vi "Instrument Manager Loop.vi"(8 "System Control":refnum<queue>, 11 "Instrument Manager":refnum<queue>) -> (0 "error out":errorcluster)   [LabVIEW 2020, in "ChromTech Next Gen Compensator Pump.lvlib" / "Instrument Manager.lvlib"]
uses:
  Instrument Manager/Instrument Manager.lvlib
  support/Message Queue/Message Cluster.ctl
  Instrument Manager/Instrument State.ctl
  <vilib>/Utility/error.llb/Error Cluster From Error Code.vi
  <vilib>/ErrorRing/Error Ring.xnode
  support/Message Queue/Message Queue.lvlib
  ChromTech Next Gen Compensator Pump.lvlib
  <instrlib>/RxnRover/ChromtechNextGenDriver/ChromTech MX-Class Drivers.lvlib
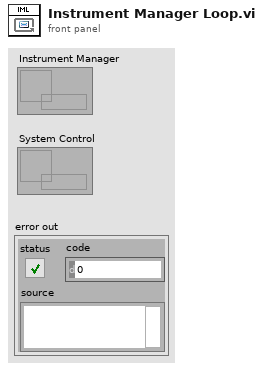
[diagram p1: front panel]
types:
  T1 = typedef "ChromTech Next Gen Compensator Pump.lvlib/Instrument Manager.lvlib/Instrument State.ctl" = cluster{"VISA Resource":refnum<visa-resource-name>, "Flow Rate":dbl, "Running":bool, "Running Since":timestamp, "Pressure Data Point":cluster{"Time Stamp":timestamp, "Value":dbl}, "Upper Pressure Fault":bool, "Lower Pressure Fault":bool, "Motor Stall Fault":bool, "Sampling Rate (sec/sample)":dbl, "Retry Attempts":i32, "Fast Comms":bool, "Total Flow Rate":dbl, "Other Flow Rate":dbl}
  T2 = cluster{"seconds since 1Jan1904":timestamp, "Pressure":dbl}
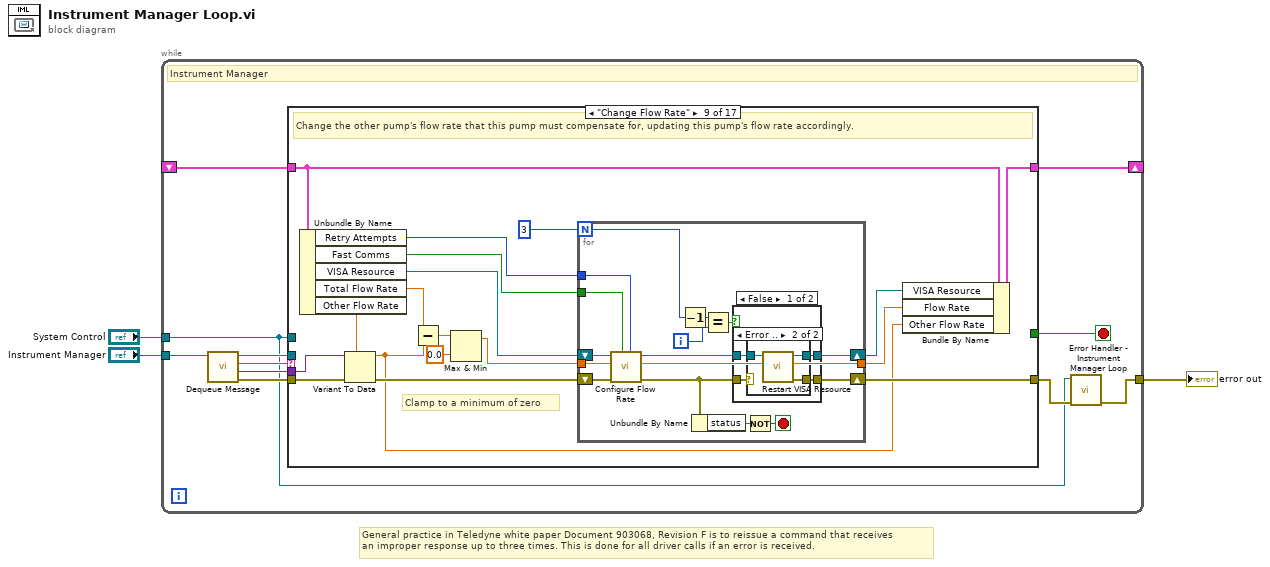
[diagram p0: block diagram]
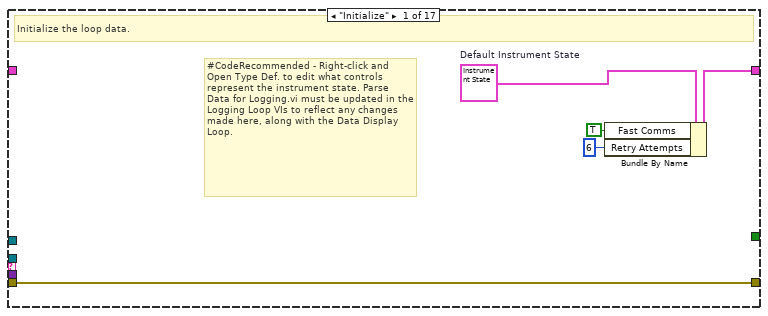
[diagram p2: hidden frame]
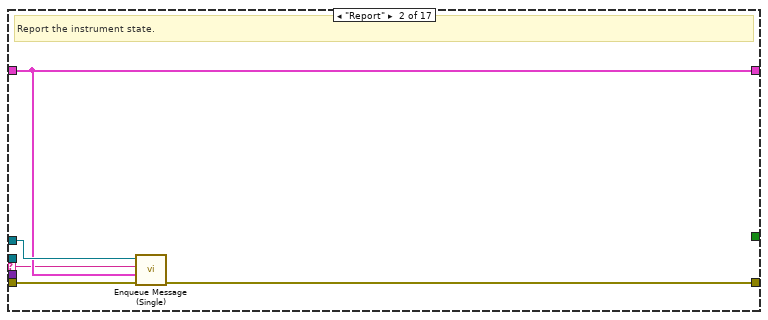
[diagram p3: hidden frame]
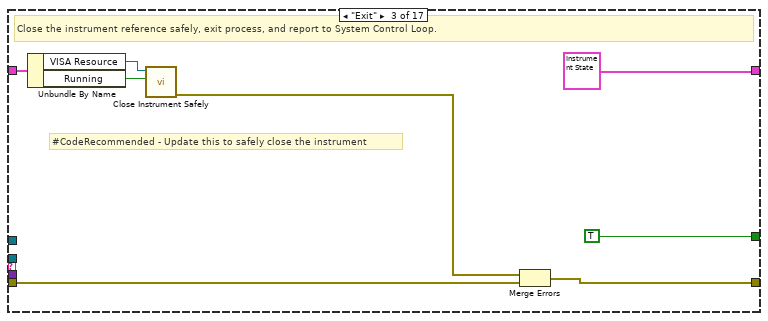
[diagram p4: hidden frame]
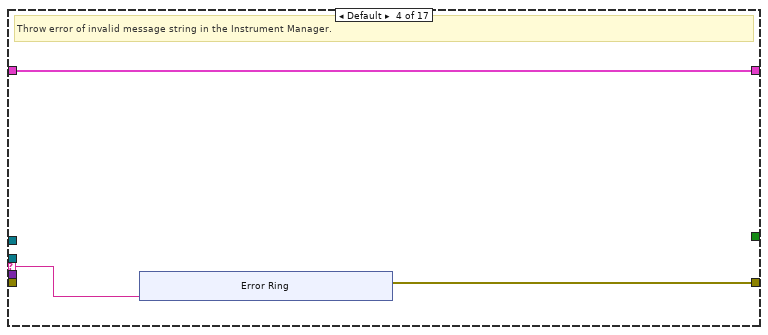
[diagram p5: hidden frame]
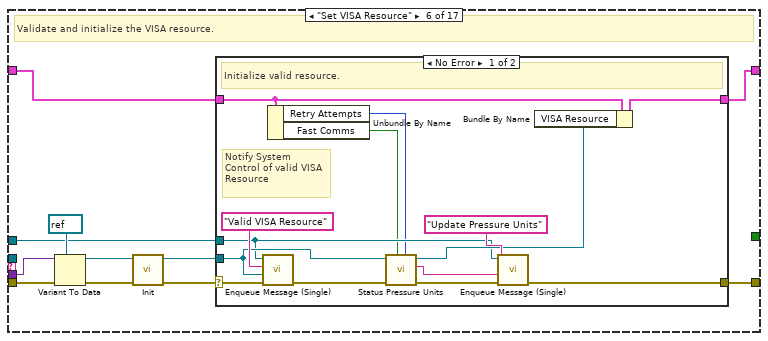
[diagram p7: hidden frame]
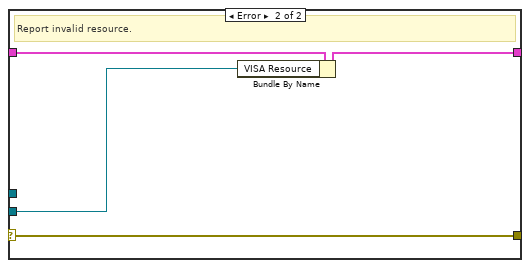
[diagram p8: hidden frame]
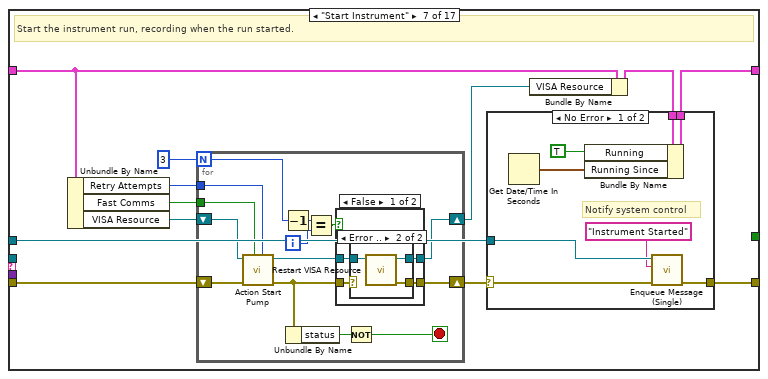
[diagram p9: hidden frame]
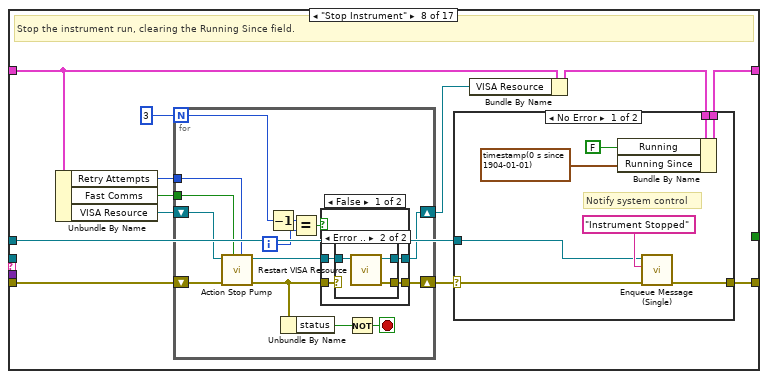
[diagram p13: hidden frame]
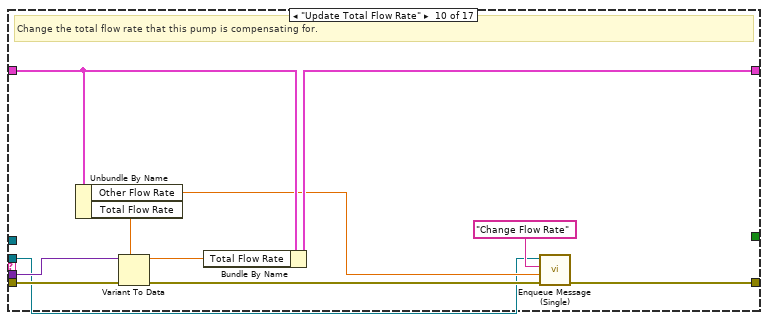
[diagram p19: hidden frame]
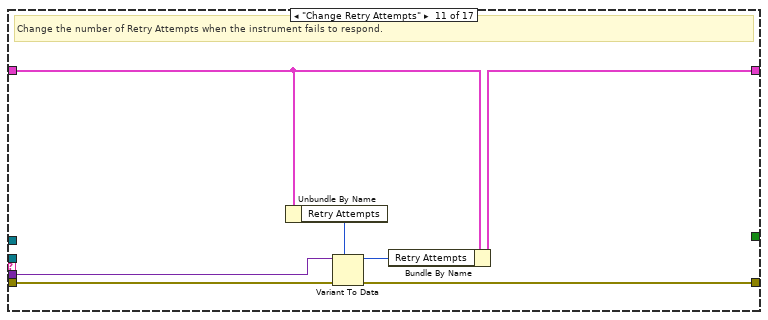
[diagram p20: hidden frame]
diagram:
  # "General practice in Teledyne white paper Document 903068, Revision F is to reissue a command that receives\nan improper response up to three times. This is done for all driver calls if an error is received."
  n1 = while {
    tunnel: "Instrument Manager" -> [w14]
    tunnel: "System Control" -> [w4]
    tunnel: [w8] -> w1
    shift-right: [w6] -> _
    shift-left: _ -> [w7]
    stop <- w5 stop-if-true
    # "Instrument Manager"
    n2 = call "Dequeue Message.vi"("Message Queue"=w14) -> ("error out"=w10:errorcluster, "Message Data"=w11:variant, "Message"=w13:string, "dup Message Queue"=w12:refnum<queue>)  [unwired: 7 in]
    n3 = case shown="\"Change Flow Rate\"" w13 {
      selector: w13 -> [_ w20 _ w34 _ _ _ _ _ _ _ _ _ _ _ _ _]
      tunnel: w12 -> [_ _ _ _ _ _ _ _ _ w213 _ _ _ _ _ _ _]
      tunnel: w4 -> [_ w23 _ _ _ w45 w84 w131 _ _ _ _ _ _ _ _ _]
      tunnel: w11 -> [_ _ _ _ _ w52 _ _ w184 w222 w229 w236 _ _ _ _ _]
      tunnel: w10 -> [w18 w24 w27 _ w43 w51 w82 w129 w175 w219 w225 w232 w240 w249 w284 w324 w365]
      tunnel: [w18 w22 w26 w33 w43 w55 w85 w132 w181 w215 w224 w231 w240 w248 w283 w322 w358] -> w9
      tunnel: w7 -> [_ w21 w32 w35 w44 w54 w81 w127 w183 w221 w228 w235 w239 w247 w285 w321 w362]
      tunnel: [w17 w21 T1 {"VISA Resource"="", "Flow Rate"=0.0, "Running"=FALSE, "Running Since"=timestamp(0 s since 1904-01-01), "Pressure Data Point"={"Time Stamp"=timestamp(0 s since 1904-01-01), "Value"=0.0}, "Upper Pressure Fault"=FALSE, "Lower Pressure Fault"=FALSE, "Motor Stall Fault"=FALSE, "Sampling Rate (sec/sample)"=0.0, "Retry Attempts"=0, "Fast Comms"=FALSE, "Total Flow Rate"=0.0, "Other Flow Rate"=0.0} w35 w44 w53 w83 w130 w185 w223 w230 w237 w239 w250 w288 w323 w364] -> w6
      tunnel: [_ _ TRUE _ _ _ _ _ _ _ _ _ _ _ _ _ _] -> w5
      frame "Initialize" {
        w19 = T1 {"VISA Resource"="", "Flow Rate"=0.0, "Running"=FALSE, "Running Since"=timestamp(0 s since 1904-01-01), "Pressure Data Point"={"Time Stamp"=timestamp(0 s since 1904-01-01), "Value"=0.0}, "Upper Pressure Fault"=FALSE, "Lower Pressure Fault"=FALSE, "Motor Stall Fault"=FALSE, "Sampling Rate (sec/sample)"=0.0, "Retry Attempts"=0, "Fast Comms"=FALSE, "Total Flow Rate"=0.0, "Other Flow Rate"=0.0}  # Default Instrument State
        # "#CodeRecommended - Right-click and Open Type Def. to edit what controls represent the instrument state. Parse Data for Logging.vi must be updated in the Logging Loop VIs to reflect any changes made here, along with the Data Display Loop."
        # "Initialize the loop data."
        n4 = Bundle By Name(cluster=w19, "Fast Comms"=TRUE, "Retry Attempts"=6) -> (w17:T1)
      }
      frame "Report" {
        # "Report the instrument state."
        n5 = call "Enqueue Message (Single).vi"("error in (no error)"=w24, "Message Data"=w21, "Message"=w20, "Message Queue"=w23) -> ("error out"=w22:errorcluster)  [unwired: 6 in, 1 out]
      }
      frame "Exit" {
        # "#CodeRecommended - Update this to safely close the instrument"
        # "Close the instrument reference safely, exit process, and report to System Control Loop."
        n6 = Unbundle By Name(w32) -> ("VISA Resource"=w30:refnum<visa-resource-name>, "Running"=w31:bool)
        n7 = call "Close Instrument Safely.vi"("Running (F)"=w31, "VISA Refnum in"=w30) -> ("error out"=w25:errorcluster)  [unwired: 9 in]
        n8 = Merge Errors(w25, w27) -> (w26:errorcluster)
      }
      frame Default {
        # "Throw error of invalid message string in the Instrument Manager."
        n9 = xnode "Error Ring"("parameter 0"=w34) -> ("error out"=w33:errorcluster)
      }
      frame "--- Copy This Frame ---" {
        # "Copy this frame and add responses to instrument specific messages."
      }
      frame "Set VISA Resource" {
        # "Validate and initialize the VISA resource."
        n10 = Variant To Data(error in=w51, type=refnum<visa-resource-name> refnum, Variant=w52) -> (data=w49:refnum<visa-resource-name>, error out=w50:errorcluster)
        n11 = call "Init.vi"("error in (no error)"=w50, "VISA resource in"=w49) -> ("error out"=w46:errorcluster, "VISA resource out"=w47:refnum<visa-resource-name>)  [unwired: 8 in]
        n12 = case shown="No Error" w46 {
          selector: w46 -> [w69 w70]
          tunnel: w47 -> [w62 w71]
          tunnel: [w64 w70] -> w55
          tunnel: w54 -> [w58 w73]
          tunnel: [w67 w72] -> w53
          tunnel: w45 -> [w60 _]
          frame No Error {
            # "Notify System Control of valid VISA Resource"
            # "Initialize valid resource."
            n13 = call "Enqueue Message (Single).vi"("error in (no error)"=w69, "Message Data"=w62, "Message"="Valid VISA Resource", "Message Queue"=w60) -> ("error out"=w66:errorcluster)  [unwired: 6 in, 1 out]
            n14 = Unbundle By Name(w58) -> ("Retry Attempts"=w57:i32, "Fast Comms"=w56:bool)
            n15 = call <instrlib>:"Status Pressure Units.vi"("Retry Attempts (0)"=w57, "Fast Comms (F)"=w56, "error in (no error)"=w66, "VISA resource name"=w62) -> ("error out"=w65:errorcluster, "Pressure Units"=w59:string, "VISA resource name out"=w61:refnum<visa-resource-name>)  [unwired: 5 in]
            n16 = call "Enqueue Message (Single).vi"("error in (no error)"=w65, "Message Data"=w59, "Message"="Update Pressure Units", "Message Queue"=w60) -> ("error out"=w64:errorcluster)  [unwired: 6 in, 1 out]
            n17 = Bundle By Name(cluster=w58, "VISA Resource"=w61) -> (w67:T1)
          }
          frame Error {
            # "Report invalid resource."
            n18 = Bundle By Name(cluster=w73, "VISA Resource"=w71) -> (w72:T1)
          }
        }
      }
      frame "Start Instrument" {
        # "Start the instrument run, recording when the run started."
        n19 = Unbundle By Name(w81) -> ("Retry Attempts"=w77:i32, "Fast Comms"=w78:bool, "VISA Resource"=w80:refnum<visa-resource-name>)
        n20 = for {
          N: 3 -> [w89]
          tunnel: w78 -> [w97]
          tunnel: w77 -> [w96]
          shift-right: [w86] -> w79
          shift-left: w82 -> [w99]
          shift-right: [w90] -> w74
          shift-left: w80 -> [w98]
          i -> [w88]
          stop <- w94 stop-if-true
          n21 = call <instrlib>:"Action Start Pump.vi"("Retry Attempts (0)"=w96, "Fast Comms (F)"=w97, "error in"=w99, "VISA resource name"=w98) -> ("error out"=w87:errorcluster, "VISA resource name out"=w91:refnum<visa-resource-name>)  [unwired: 6 in]
          n22 = Decrement(x=w89) -> (x-1=w93:i32)
          n23 = Unbundle By Name(w87) -> ("status"=w95:bool)
          n24 = Equal?(x=w93, y=w88) -> (x = y?=w92:bool)
          n25 = case shown="False" w92 {
            tunnel: [w103 w110] -> w86
            tunnel: w91 -> [w102 w109]
            tunnel: w87 -> [w101 w110]
            tunnel: [w100 w109] -> w90
            frame False {
              n26 = case shown="Error .." w101 {
                selector: w101 -> [w105 _]
                tunnel: [w105 w108] -> w103
                tunnel: w102 -> [w104 w107]
                tunnel: [w104 w106] -> w100
                frame No Error {
                }
                frame Error {
                  n27 = call "Restart VISA Resource.vi"("VISA Refnum in"=w107) -> ("error out"=w108:errorcluster, "VISA resource name out"=w106:refnum<visa-resource-name>)  [unwired: 9 in]
                }
              }
            }
            frame True {
            }
          }
          n28 = Not(x=w95) -> (.not. x?=w94:bool)
        }
        n29 = Bundle By Name(cluster=w81, "VISA Resource"=w74) -> (w75:T1)
        n30 = case shown="No Error" w79 {
          selector: w79 -> [w111 w120]
          tunnel: [w118 w120] -> w85
          tunnel: w84 -> [w117 _]
          tunnel: [w115 w119] -> w83
          tunnel: w75 -> [w112 w119]
          frame No Error {
            # "Notify system control"
            n31 = Get Date/Time In Seconds() -> (seconds since 1Jan1904=w113:timestamp)
            n32 = Bundle By Name(cluster=w112, "Running"=TRUE, "Running Since"=w113) -> (w115:T1)
            n33 = call "Enqueue Message (Single).vi"("error in (no error)"=w111, "Message"="Instrument Started", "Message Queue"=w117) -> ("error out"=w118:errorcluster)  [unwired: 7 in, 1 out]
          }
          frame Error {
          }
        }
      }
      frame "Stop Instrument" {
        # "Stop the instrument run, clearing the Running Since field."
        n34 = Unbundle By Name(w127) -> ("Retry Attempts"=w124:i32, "Fast Comms"=w125:bool, "VISA Resource"=w126:refnum<visa-resource-name>)
        n35 = for {
          N: 3 -> [w135]
          tunnel: w125 -> [w144]
          tunnel: w124 -> [w143]
          shift-right: [w136] -> w128
          shift-left: w129 -> [w146]
          shift-right: [w138] -> w121
          shift-left: w126 -> [w145]
          i -> [w134]
          stop <- w141 stop-if-true
          n36 = call <instrlib>:"Action Stop Pump.vi"("Retry Attempts (0)"=w143, "Fast Comms (F)"=w144, "error in"=w146, "VISA resource name"=w145) -> ("error out"=w137:errorcluster, "VISA resource name out"=w139:refnum<visa-resource-name>)  [unwired: 6 in]
          n37 = Decrement(x=w135) -> (x-1=w140:i32)
          n38 = Unbundle By Name(w137) -> ("status"=w142:bool)
          n39 = Equal?(x=w140, y=w134) -> (x = y?=w133:bool)
          n40 = case shown="False" w133 {
            tunnel: [w150 w157] -> w136
            tunnel: w139 -> [w149 w156]
            tunnel: w137 -> [w148 w157]
            tunnel: [w147 w156] -> w138
            frame False {
              n41 = case shown="Error .." w148 {
                selector: w148 -> [w152 _]
                tunnel: [w152 w155] -> w150
                tunnel: w149 -> [w151 w154]
                tunnel: [w151 w153] -> w147
                frame No Error {
                }
                frame Error {
                  n42 = call "Restart VISA Resource.vi"("VISA Refnum in"=w154) -> ("error out"=w155:errorcluster, "VISA resource name out"=w153:refnum<visa-resource-name>)  [unwired: 9 in]
                }
              }
            }
            frame True {
            }
          }
          n43 = Not(x=w142) -> (.not. x?=w141:bool)
        }
        n44 = Bundle By Name(cluster=w127, "VISA Resource"=w121) -> (w122:T1)
        n45 = case shown="No Error" w128 {
          selector: w128 -> [w158 w167]
          tunnel: w122 -> [w165 w166]
          tunnel: [w164 w167] -> w132
          tunnel: w131 -> [w162 _]
          tunnel: [w161 w166] -> w130
          frame No Error {
            # "Notify system control"
            n46 = Bundle By Name(cluster=w165, "Running"=FALSE, "Running Since"=timestamp(0 s since 1904-01-01)) -> (w161:T1)
            n47 = call "Enqueue Message (Single).vi"("error in (no error)"=w158, "Message"="Instrument Stopped", "Message Queue"=w162) -> ("error out"=w164:errorcluster)  [unwired: 7 in, 1 out]
          }
          frame Error {
          }
        }
      }
      frame "Change Flow Rate" {
        # "Clamp to a minimum of zero"
        # "Change the other pump's flow rate that this pump must compensate for, updating this pump's flow rate accordingly."
        n48 = Unbundle By Name(w183) -> ("Retry Attempts"=w179:i32, "Fast Comms"=w178:bool, "VISA Resource"=w182:refnum<visa-resource-name>, "Total Flow Rate"=w172:dbl, "Other Flow Rate"=w173:dbl)
        n49 = Variant To Data(error in=w175, type=w173, Variant=w184) -> (data=w168:dbl, error out=w174:errorcluster)
        n50 = Subtract(x=w172, y=w168) -> (x-y=w170:dbl)
        n51 = Max & Min(x=w170, y=0.0) -> (max(x,y)=w169:dbl)  [unwired: 1 out]
        n52 = for {
          N: 3 -> [w188]
          tunnel: w169 -> [w200]
          tunnel: [w199] -> w180
          tunnel: w179 -> [w198]
          tunnel: w178 -> [w197]
          shift-right: [w191] -> w181
          shift-left: w174 -> [w196]
          shift-right: [w189] -> w176
          shift-left: w182 -> [w201]
          i -> [w187]
          stop <- w194 stop-if-true
          n53 = call <instrlib>:"Configure Flow Rate.vi"("Retry Attempts (0)"=w198, "Fast Comms (F)"=w197, "error in"=w196, "Flow Input (ml/min)"=w200, "VISA resource name"=w201) -> ("error out"=w192:errorcluster, "Flow Output"=w199:dbl, "VISA resource name out"=w190:refnum<visa-resource-name>)  [unwired: 4 in]
          n54 = Decrement(x=w188) -> (x-1=w193:i32)
          n55 = Unbundle By Name(w192) -> ("status"=w195:bool)
          n56 = Equal?(x=w193, y=w187) -> (x = y?=w186:bool)
          n57 = case shown="False" w186 {
            tunnel: [w205 w212] -> w191
            tunnel: w190 -> [w204 w211]
            tunnel: w192 -> [w203 w212]
            tunnel: [w202 w211] -> w189
            frame False {
              n58 = case shown="Error .." w203 {
                selector: w203 -> [w207 _]
                tunnel: [w207 w210] -> w205
                tunnel: w204 -> [w206 w209]
                tunnel: [w206 w208] -> w202
                frame No Error {
                }
                frame Error {
                  n59 = call "Restart VISA Resource.vi"("VISA Refnum in"=w209) -> ("error out"=w210:errorcluster, "VISA resource name out"=w208:refnum<visa-resource-name>)  [unwired: 9 in]
                }
              }
            }
            frame True {
            }
          }
          n60 = Not(x=w195) -> (.not. x?=w194:bool)
        }
        n61 = Bundle By Name(cluster=w183, "VISA Resource"=w176, "Flow Rate"=w180, "Other Flow Rate"=w168) -> (w185:T1)
      }
      frame "Update Total Flow Rate" {
        # "Change the total flow rate that this pump is compensating for."
        n62 = Unbundle By Name(w221) -> ("Other Flow Rate"=w214:dbl, "Total Flow Rate"=w220:dbl)
        n63 = Variant To Data(error in=w219, type=w220, Variant=w222) -> (data=w218:dbl, error out=w216:errorcluster)
        n64 = Bundle By Name(cluster=w221, "Total Flow Rate"=w218) -> (w223:T1)
        n65 = call "Enqueue Message (Single).vi"("error in (no error)"=w216, "Message Data"=w214, "Message"="Change Flow Rate", "Message Queue"=w213) -> ("error out"=w215:errorcluster)  [unwired: 6 in, 1 out]
      }
      frame "Change Retry Attempts" {
        # "Change the number of Retry Attempts when the instrument fails to respond."
        n66 = Unbundle By Name(w228) -> ("Retry Attempts"=w226:i32)
        n67 = Variant To Data(error in=w225, type=w226, Variant=w229) -> (data=w227:i32, error out=w224:errorcluster)
        n68 = Bundle By Name(cluster=w228, "Retry Attempts"=w227) -> (w230:T1)
      }
      frame "Change Fast Comms" {
        # "Change whether to use a return character ('\\r', 0x0D) at the end of each message to the pump. The return character will terminate the write commands to avoid delays by the pump waiting for partial commands."
        n69 = Unbundle By Name(w235) -> ("Fast Comms"=w233:bool)
        n70 = Variant To Data(error in=w232, type=w233, Variant=w236) -> (data=w234:bool, error out=w231:errorcluster)
        n71 = Bundle By Name(cluster=w235, "Fast Comms"=w234) -> (w237:T1)
      }
      frame "--- Copy for Get State Messages ---" {
        # "Wait 100 ms because if two commands are sent in quick succession, the second will fail."
        # "#CodeNeeded - Use the Bundle by Name function to bundle the new state value into the Instrument State cluster."
        # "#CodeNeeded - Add instrument driver call to query the instrument state requested"
        # "Duplicate this case for messages cases that will query the instrument state."
        n72 = Wait (ms)(milliseconds to wait=u32 100) -> ()  [unwired: 1 out]
      }
      frame "Run State" {
        # "Query the run state of the instrument."
        n73 = Unbundle By Name(w247) -> ("Retry Attempts"=w244:i32, "Fast Comms"=w243:bool, "VISA Resource"=w246:refnum<visa-resource-name>)
        n74 = for {
          N: 3 -> [w252]
          tunnel: [w264] -> w245
          tunnel: w244 -> [w263]
          tunnel: w243 -> [w262]
          shift-right: [w256] -> w248
          shift-left: w249 -> [w261]
          shift-right: [w254] -> w241
          shift-left: w246 -> [w265]
          i -> [w253]
          stop <- w259 stop-if-true
          n75 = call <instrlib>:"Status Run State.vi"("Retry Attempts (0)"=w263, "Fast Comms (F)"=w262, "error in (no error)"=w261, "VISA resource name"=w265) -> ("error out"=w257:errorcluster, "Running?"=w264:bool, "VISA resource name out"=w255:refnum<visa-resource-name>)  [unwired: 5 in]
          n76 = Decrement(x=w252) -> (x-1=w258:i32)
          n77 = Unbundle By Name(w257) -> ("status"=w260:bool)
          n78 = Equal?(x=w258, y=w253) -> (x = y?=w251:bool)
          n79 = case shown="False" w251 {
            tunnel: [w269 w276] -> w256
            tunnel: w255 -> [w268 w275]
            tunnel: w257 -> [w267 w276]
            tunnel: [w266 w275] -> w254
            frame False {
              n80 = case shown="Error .." w267 {
                selector: w267 -> [w271 _]
                tunnel: [w271 w274] -> w269
                tunnel: w268 -> [w270 w273]
                tunnel: [w270 w272] -> w266
                frame No Error {
                }
                frame Error {
                  n81 = call "Restart VISA Resource.vi"("VISA Refnum in"=w273) -> ("error out"=w274:errorcluster, "VISA resource name out"=w272:refnum<visa-resource-name>)  [unwired: 9 in]
                }
              }
            }
            frame True {
            }
          }
          n82 = Not(x=w260) -> (.not. x?=w259:bool)
        }
        n83 = Bundle By Name(cluster=w247, "VISA Resource"=w241, "Running"=w245) -> (w250:T1)
      }
      frame "Pressure" {
        # "Query the pressure value of the instrument."
        n84 = Unbundle By Name(w285) -> ("Retry Attempts"=w279:i32, "Fast Comms"=w280:bool, "VISA Resource"=w282:refnum<visa-resource-name>)
        n85 = for {
          N: 3 -> [w290]
          tunnel: [w302] -> w281
          tunnel: w280 -> [w301]
          tunnel: w279 -> [w300]
          shift-right: [w294] -> w283
          shift-left: w284 -> [w299]
          shift-right: [w292] -> w277
          shift-left: w282 -> [w303]
          i -> [w291]
          stop <- w297 stop-if-true
          n86 = call <instrlib>:"Status Get Pressure.vi"("Retry Attempts (0)"=w300, "Fast Comms (F)"=w301, "error in"=w299, "VISA resource name"=w303) -> ("error out"=w295:errorcluster, "Pressure"=w302:dbl, "VISA resource name out"=w293:refnum<visa-resource-name>)  [unwired: 5 in]
          n87 = Decrement(x=w290) -> (x-1=w296:i32)
          n88 = Unbundle By Name(w295) -> ("status"=w298:bool)
          n89 = Equal?(x=w296, y=w291) -> (x = y?=w289:bool)
          n90 = case shown="False" w289 {
            tunnel: [w307 w314] -> w294
            tunnel: w293 -> [w306 w313]
            tunnel: w295 -> [w305 w314]
            tunnel: [w304 w313] -> w292
            frame False {
              n91 = case shown="Error .." w305 {
                selector: w305 -> [w309 _]
                tunnel: [w309 w312] -> w307
                tunnel: w306 -> [w308 w311]
                tunnel: [w308 w310] -> w304
                frame No Error {
                }
                frame Error {
                  n92 = call "Restart VISA Resource.vi"("VISA Refnum in"=w311) -> ("error out"=w312:errorcluster, "VISA resource name out"=w310:refnum<visa-resource-name>)  [unwired: 9 in]
                }
              }
            }
            frame True {
            }
          }
          n93 = Not(x=w298) -> (.not. x?=w297:bool)
        }
        n94 = Get Date/Time In Seconds() -> (seconds since 1Jan1904=w287:timestamp)
        n95 = Bundle("seconds since 1Jan1904"=w287, "Pressure"=w281) -> (w286:T2)  [unwired: 1 in]
        n96 = Bundle By Name(cluster=w285, "Pressure Data Point"=w286, "VISA Resource"=w277) -> (w288:T1)
      }
      frame "Flow Rate" {
        # "Query the flow rate of the instrument."
        n97 = Unbundle By Name(w321) -> ("Retry Attempts"=w318:i32, "Fast Comms"=w317:bool, "VISA Resource"=w320:refnum<visa-resource-name>)
        n98 = for {
          N: 3 -> [w328]
          tunnel: [w338] -> w319
          tunnel: w318 -> [w337]
          tunnel: w317 -> [w336]
          shift-right: [w330] -> w322
          shift-left: w324 -> [w335]
          shift-right: [w325] -> w315
          shift-left: w320 -> [w339]
          i -> [w327]
          stop <- w333 stop-if-true
          n99 = call <instrlib>:"Status Get Flow Rate.vi"("Retry Attempts (0)"=w337, "Fast Comms (F)"=w336, "error in"=w335, "VISA resource name"=w339) -> ("error out"=w331:errorcluster, "Flow Rate"=w338:dbl, "VISA resource name out"=w326:refnum<visa-resource-name>)  [unwired: 5 in]
          n100 = Unbundle By Name(w331) -> ("status"=w334:bool)
          n101 = Decrement(x=w328) -> (x-1=w332:i32)
          n102 = Equal?(x=w332, y=w327) -> (x = y?=w329:bool)
          n103 = case shown="False" w329 {
            tunnel: [w343 w350] -> w330
            tunnel: w326 -> [w342 w349]
            tunnel: w331 -> [w341 w350]
            tunnel: [w340 w349] -> w325
            frame False {
              n104 = case shown="Error .." w341 {
                selector: w341 -> [w345 _]
                tunnel: [w345 w348] -> w343
                tunnel: w342 -> [w344 w347]
                tunnel: [w344 w346] -> w340
                frame No Error {
                }
                frame Error {
                  n105 = call "Restart VISA Resource.vi"("VISA Refnum in"=w347) -> ("error out"=w348:errorcluster, "VISA resource name out"=w346:refnum<visa-resource-name>)  [unwired: 9 in]
                }
              }
            }
            frame True {
            }
          }
          n106 = Not(x=w334) -> (.not. x?=w333:bool)
        }
        n107 = Bundle By Name(cluster=w321, "VISA Resource"=w315, "Flow Rate"=w319) -> (w323:T1)
      }
      frame "Faults" {
        # "Query the fault status of the instrument."
        n108 = Unbundle By Name(w362) -> ("Retry Attempts"=w354:i32, "Fast Comms"=w353:bool, "VISA Resource"=w361:refnum<visa-resource-name>)
        n109 = for {
          N: 3 -> [w368]
          tunnel: [w380] -> w360
          tunnel: [w379] -> w359
          tunnel: [w378] -> w355
          tunnel: w354 -> [w377]
          tunnel: w353 -> [w376]
          shift-right: [w371] -> w363
          shift-left: w365 -> [w382]
          shift-right: [w369] -> w351
          shift-left: w361 -> [w381]
          i -> [w367]
          stop <- w374 stop-if-true
          n110 = call <instrlib>:"Status Faults.vi"("VISA resource name"=w381, "Fast Comms (F)"=w376, "Retry Attempts (0)"=w377, "error in (no error)"=w382) -> ("VISA resource name out"=w370:refnum<visa-resource-name>, "Upper Pressure Fault"=w379:bool, "Lower Pressure Fault"=w380:bool, "Motor Stall Fault"=w378:bool, "error out"=w372:errorcluster)  [unwired: 7 in]
          n111 = Decrement(x=w368) -> (x-1=w373:i32)
          n112 = Unbundle By Name(w372) -> ("status"=w375:bool)
          n113 = Equal?(x=w373, y=w367) -> (x = y?=w366:bool)
          n114 = Not(x=w375) -> (.not. x?=w374:bool)
          n115 = case shown="False" w366 {
            tunnel: [w386 w393] -> w371
            tunnel: w370 -> [w385 w392]
            tunnel: w372 -> [w384 w393]
            tunnel: [w383 w392] -> w369
            frame False {
              n116 = case shown="Error .." w384 {
                selector: w384 -> [w388 _]
                tunnel: [w388 w391] -> w386
                tunnel: w385 -> [w387 w390]
                tunnel: [w387 w389] -> w383
                frame No Error {
                }
                frame Error {
                  n117 = call "Restart VISA Resource.vi"("VISA Refnum in"=w390) -> ("error out"=w391:errorcluster, "VISA resource name out"=w389:refnum<visa-resource-name>)  [unwired: 9 in]
                }
              }
            }
            frame True {
            }
          }
        }
        n118 = Build Array(w355, w360, w359) -> (w356:bool[])
        n119 = Bundle By Name(cluster=w362, "VISA Resource"=w351, "Upper Pressure Fault"=w359, "Lower Pressure Fault"=w360, "Motor Stall Fault"=w355) -> (w364:T1)
        n120 = Or Array Elements(Boolean array=w356) -> (logical OR=w357:bool)
        n121 = case shown="True" w357 {
          tunnel: w363 -> [w394 w398]
          tunnel: [w394 w397] -> w358
          tunnel: w356 -> [_ w395]
          frame False {
          }
          frame True {
            n122 = call "Error Cluster from Fault.vi"("Fault indicators"=w395) -> ("error out"=w396:errorcluster)  [unwired: 10 in]
            n123 = Merge Errors(w396, w398) -> (w397:errorcluster)
          }
        }
      }
    }
    n124 = call "Error Handler - Instrument Manager Loop.vi"("error in (no error)"=w9, "Message Queue"=w4) -> ("dup error in"=w8:errorcluster)  [unwired: 8 in, 1 out]
  }
  "error out" <- w1
